vi "tra25cc_close.vi"(8 "error in (no error)":errorcluster, 11 "conn_xyz_in":T1) -> (0 "error out":errorcluster)   [LabVIEW 2018]
uses:
  D:/Data/Thea/tests/Labview/Scanner_v3_Phy-2019.05.06/src/Stage_xyz/Dll/Newport.CONEXCC.CommandInterface.dll
  Dll/Newport.CONEXCC.CommandInterface.dll
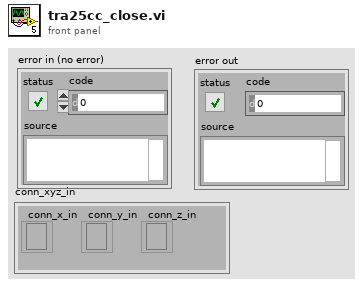
[diagram p1: front panel]
types:
  T1 = cluster{"conn_x_in":refnum<k24>, "conn_y_in":refnum<k24>, "conn_z_in":refnum<k24>}
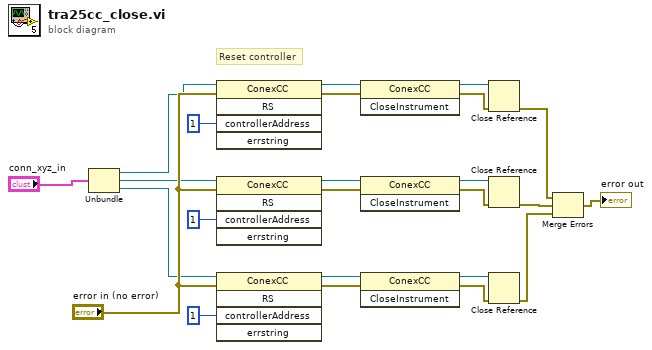
[diagram p0: block diagram]
diagram:
  # "Reset controller"
  n1 = Unbundle("conn_xyz_in") -> ("conn_x_in"=w3:refnum<k24>, "conn_y_in"=w2:refnum<k24>, "conn_z_in"=w1:refnum<k24>)
  n2 = invoke class="ConexCC" method="RS"(reference=w3, error in="error in (no error)", "controllerAddress"=1) -> (reference out=w24:refnum<k24>, error out=w23:errorcluster)  [unwired: 2 in, 3 out]
  n3 = invoke class="ConexCC" method="RS"(reference=w2, error in="error in (no error)", "controllerAddress"=1) -> (reference out=w19:refnum<k24>, error out=w18:errorcluster)  [unwired: 2 in, 3 out]
  n4 = invoke class="ConexCC" method="RS"(reference=w1, error in="error in (no error)", "controllerAddress"=1) -> (reference out=w14:refnum<k24>, error out=w13:errorcluster)  [unwired: 2 in, 3 out]
  n5 = invoke class="ConexCC" method="CloseInstrument"(reference=w24, error in=w23) -> (reference out=w20:refnum<k24>, error out=w21:errorcluster)  [unwired: 1 in, 1 out]
  n6 = invoke class="ConexCC" method="CloseInstrument"(reference=w19, error in=w18) -> (reference out=w15:refnum<k24>, error out=w16:errorcluster)  [unwired: 1 in, 1 out]
  n7 = invoke class="ConexCC" method="CloseInstrument"(reference=w14, error in=w13) -> (reference out=w10:refnum<k24>, error out=w11:errorcluster)  [unwired: 1 in, 1 out]
  n8 = Close Reference(reference=w20, error in (no error)=w21) -> (error out=w7:errorcluster)
  n9 = Close Reference(reference=w15, error in (no error)=w16) -> (error out=w9:errorcluster)
  n10 = Close Reference(reference=w10, error in (no error)=w11) -> (error out=w8:errorcluster)
  n11 = Merge Errors(w7, w9, w8) -> (→"error out":errorcluster)
